vi "CaseStructureUnderStanding.vi"() -> ()   [LabVIEW 2019]
panel:
  out "Temprature in celsisus":dbl
  in  "Boolean":bool
  in  "Temp in Farenhit":dbl(slide) scale=0.0..100.0
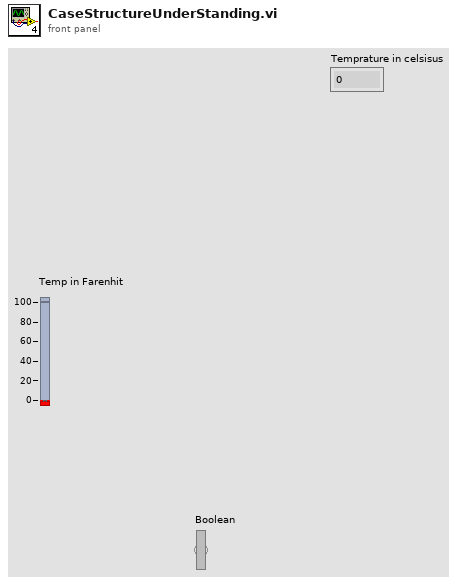
[diagram p1: front panel]
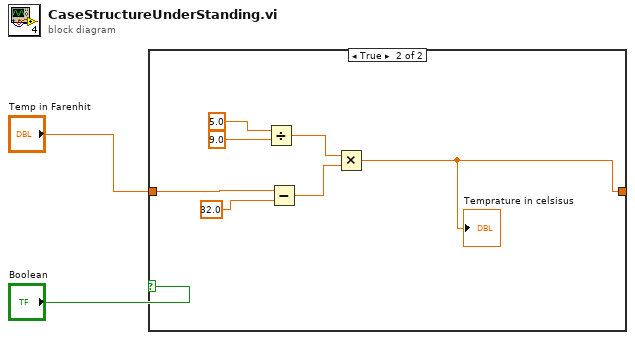
[diagram p0: block diagram]
diagram:
  n1 = case shown="True" "Boolean" {
    tunnel: "Temp in Farenhit" -> [w3 w8]
    tunnel: [w3 w4] -> _
    frame False {
    }
    frame True {
      n2 = Divide(x=5.0, y=9.0) -> (x/y=w6:dbl)
      n3 = Subtract(x=w8, y=32.0) -> (x-y=w5:dbl)
      n4 = Multiply(x=w6, y=w5) -> (x*y=w4:dbl)
      "Temprature in celsisus" <- w4
    }
  }
